vi "NewAutoWriteFile.vi"(9 "Array":T1[](array[typedef]), 10 "Comment":string, 11 "Trajectory File Name":path) -> (0 "error out":errorcluster)   [LabVIEW 2023]
doc: "Create a CSV file from a Trajectory data structure. This can be used on a PC or the RoboRIO.\n\nParameters:\n - Trajectory - Data structure containing trajectory\n - TrajectoryConfig - Trajectory configuration\n - Trajectory File Name - File name to write to. Existing files are overwritten.\n - Comment - Comment string to include in file comments.\n - Waypoints - waypoints to include in file comments\n - TrajectoryIsRelative - Relative if TRUE otherwise absolute\n - TrajectoryIsCubic - Cubic if TRUE otherwise Quintic\n\nReturns:\n - Error out - returned error cluster\n\nReturns:\n - outTrajectory - Trajectory data structure\n - Error out - returned error cluster"
uses:
  NewAutoStepTypedef.ctl
  NewAutoStepTypeEnum.ctl
  <vilib>/Rock Robotics/WPI/ThirdParty/JAS_Junk/TrajLib/Trajectory_Library.lvlib
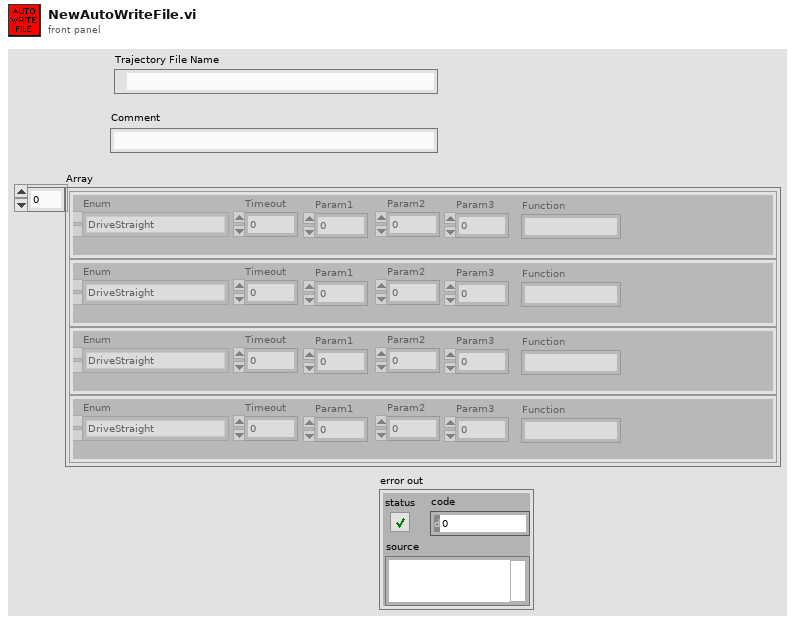
[diagram p1: front panel]
types:
  T1 = typedef "NewAutoStepTypedef.ctl" = cluster{"Enum":T2, "Timeout":dbl, "Param1":dbl, "Param2":dbl, "Param3":dbl, "Function":string}
  T2 = typedef "NewAutoStepTypeEnum.ctl" = enum16{"DriveStraight", "DriveTurn", "FollowAbsoluteTrajectory", "FollowRelativeTrajectory", "AutoWait", "ElevToRest", "ElevToFloor", "ElevToSource", "ElevToL1", "ElevToL2", "ElevToL3", "ElevToL4", "ElevToAlgae1", "ElevToAlgae2", "ElevToBarge", "ElevCancel", "IntakeCoral", "IntakeAlgae", "IntakeDepositCoral", "IntakeDepositAlgae", "IntakeCancel", "ElevRestWait", "ElevFloorWait", "ElevSourceWait", "ElevL1Wait", "ElevL2Wait", "ElevAlgae1Wait", "ElevL3Wait", "ElevAlgae2Wait", "ElevL4Wait", "ElevBargeWait"}
  T3 = enum16{"open", "replace", "create", "open or create", "replace or create", "replace or create with confirmation"}
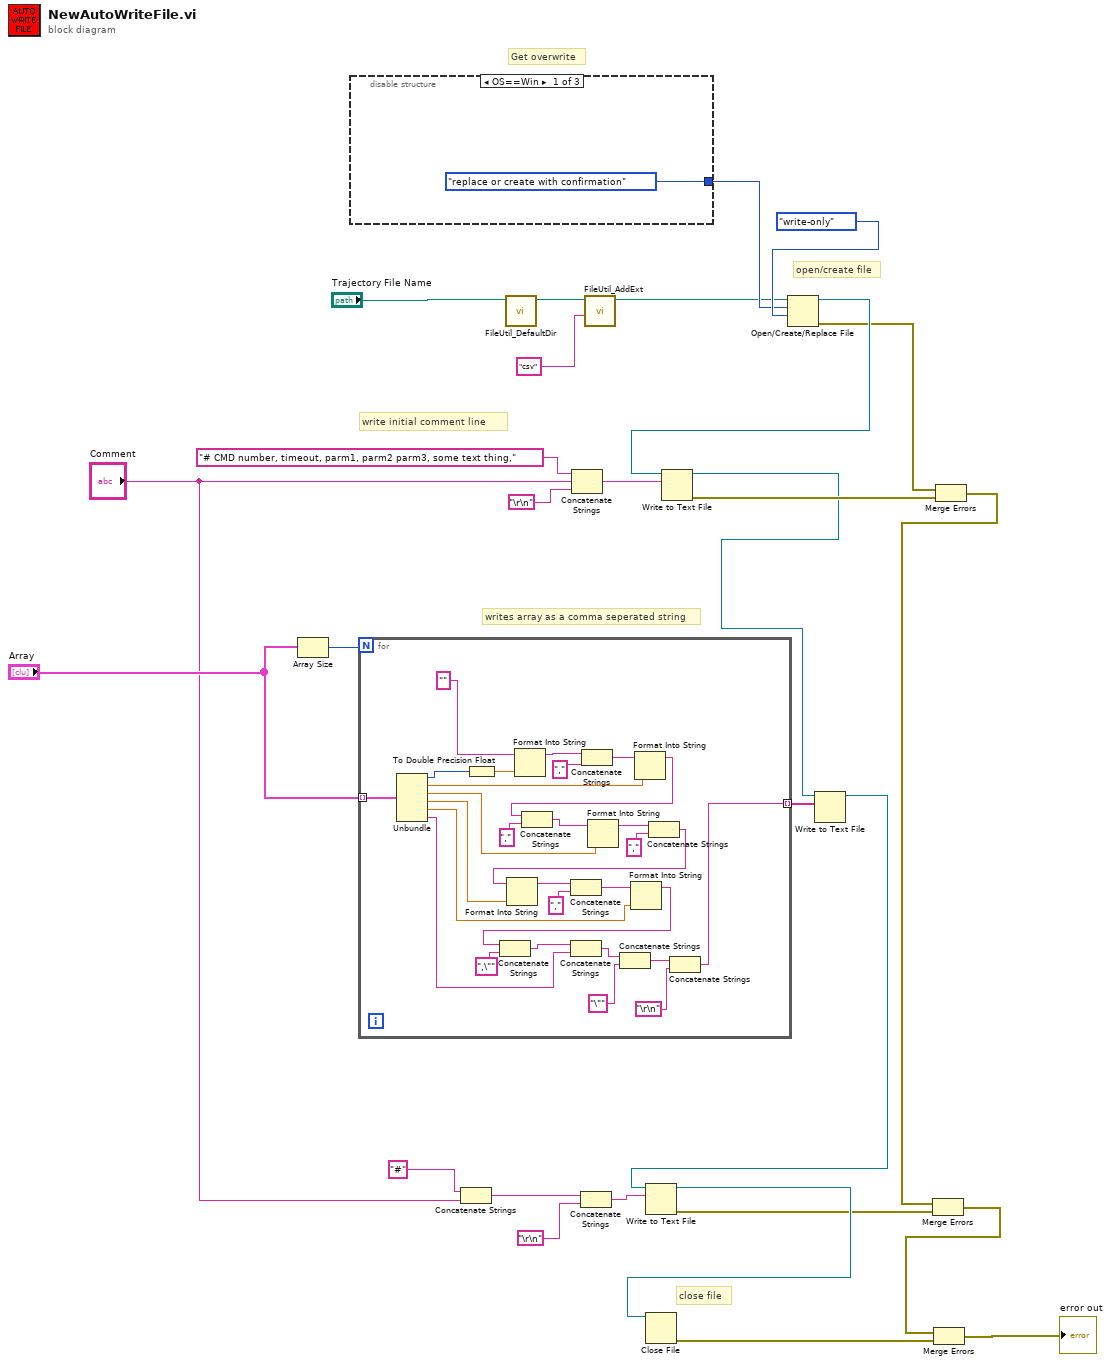
[diagram p0: block diagram]
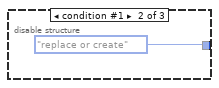
[diagram p2: hidden frame]
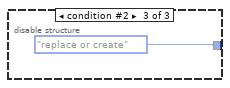
[diagram p3: hidden frame]
diagram:
  # "writes array as a comma seperated string"
  # "Get overwrite"
  # "open/create file"
  # "close file"
  # "write initial comment line"
  n1 = Array Size(array="Array") -> (size(s)=w8:i32)
  n2 = disable-structure shown="OS==Win" {
    disable-tunnel: [T3."replace or create with confirmation" ("operation (0:open)") T3."replace or create" ("operation (0:open)") T3."replace or create" ("operation (0:open)")] -> w14
    frame condition #0 (active) {
    }
    frame condition #1 {
    }
    frame condition #2 {
    }
  }
  n3 = for {
    N: w8 -> [_]
    tunnel: "Array" -> [w60] mode=indexing
    tunnel: [w32] -> w1 mode=indexing
    n4 = Unbundle(w60) -> ("Enum"=w59:T2, "Timeout"=w53:dbl, "Param1"=w49:dbl, "Param2"=w45:dbl, "Param3"=w41:dbl, "Function"=w33:string)
    n5 = To Double Precision Float(number=w59) -> (double precision float=w57:dbl)
    n6 = Format Into String(initial string="", w57) -> (resulting string=w56:string)  [unwired: 2 in, 1 out]
    n7 = Concatenate Strings(w56, ",") -> (w54:string)
    n8 = Format Into String(initial string=w54, w53) -> (resulting string=w52:string)  [unwired: 2 in, 1 out]
    n9 = Concatenate Strings(w52, ",") -> (w50:string)
    n10 = Format Into String(initial string=w50, w49) -> (resulting string=w47:string)  [unwired: 2 in, 1 out]
    n11 = Concatenate Strings(w47, ",") -> (w46:string)
    n12 = Format Into String(initial string=w46, w45) -> (resulting string=w43:string)  [unwired: 2 in, 1 out]
    n13 = Concatenate Strings(w43, ",") -> (w42:string)
    n14 = Format Into String(initial string=w42, w41) -> (resulting string=w39:string)  [unwired: 2 in, 1 out]
    n15 = Concatenate Strings(w39, ",\"") -> (w38:string)
    n16 = Concatenate Strings(w38, w33) -> (w36:string)
    n17 = Concatenate Strings(w36, "\"") -> (w34:string)
    n18 = Concatenate Strings(w34, "\r\n") -> (w32:string)
  }
  n19 = Concatenate Strings("#", "Comment") -> (w6:string)
  n20 = call <vilib>:"FileUtil_DefaultDir.vi"("Path in"="Trajectory File Name") -> ("Path Out"=w13:path)  [unwired: 10 in]
  n21 = Concatenate Strings("# CMD number, timeout, parm1, parm2 parm3, some text thing," ("string"), "Comment", "\r\n") -> (w27:string)
  n22 = Concatenate Strings(w6, "\r\n") -> (w24:string)
  n23 = call <vilib>:"FileUtil_AddExt.vi"("Extension"="csv", "Path in"=w13) -> ("Path out"=w10:path)  [unwired: 9 in]
  n24 = Open/Create/Replace File(file path (use dialog)=w10, operation (0:open)=w14, access (0:read/write)=enum16{"read/write", "read-only", "write-only"}."write-only") -> (refnum out=w22:refnum<file>, error out=w19:errorcluster)  [unwired: 3 in, 1 out]
  n25 = Write to Text File(file (use dialog)=w22, text=w27) -> (refnum out=w2:refnum<file>, error out=w20:errorcluster)  [unwired: 2 in, 1 out]
  n26 = Write to Text File(file (use dialog)=w2, text=w1) -> (refnum out=w3:refnum<file>)  [unwired: 2 in, 2 out]
  n27 = Write to Text File(file (use dialog)=w3, text=w24) -> (refnum out=w21:refnum<file>, error out=w18:errorcluster)  [unwired: 2 in, 1 out]
  n28 = Close File(refnum=w21) -> (error out=w17:errorcluster)  [unwired: 1 in, 1 out]
  n29 = Merge Errors(w19, w20) -> (w9:errorcluster)
  n30 = Merge Errors(w9, w18) -> (w16:errorcluster)
  n31 = Merge Errors(w16, w17) -> (→"error out":errorcluster)
